vi "Range test.vi"() -> ()   [LabVIEW 2019]
uses:
  <userlib>/Agilent34410A/Agilent34410A DMM_Func.ctl
panel:
  out "Function Range Out":u16(ring) items=["100 mV", "1 V", "10 V", "100 V", "1000 V", "Min", "Max", "Def"]
  in  "error in (no error)":errorcluster
  out "Range Value":dbl
  out "Autorange":bool
  out "ChaineRep":string caption="Chaîne de réponse"
  in  "Set":bool
  out "ChaineCom":string caption="Chaîne de commande"
  in  "Function Range":u16(ring) items=["100 Ohms", "1 kOhms", "10 kOhms", "100 kOhms", "1 MOhms", "10 MOhms", "100 MOhms", "1 GOhms", "Min", "Max", "Def"]
  in  "DMM Function":T1
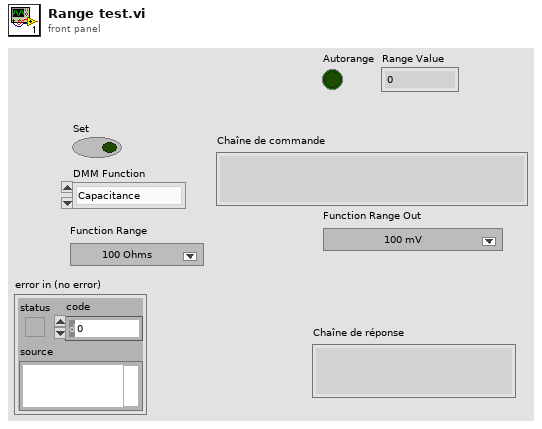
[diagram p1: front panel]
types:
  T1 = typedef "Agilent34410A DMM_Func.ctl" = enum16{"Capacitance", "Continuity", "Current AC", "Current", "Diode", "Frequency", "4W Resistance", "Period", "Resistance", "Temperature", "Voltage AC", "Voltage"}
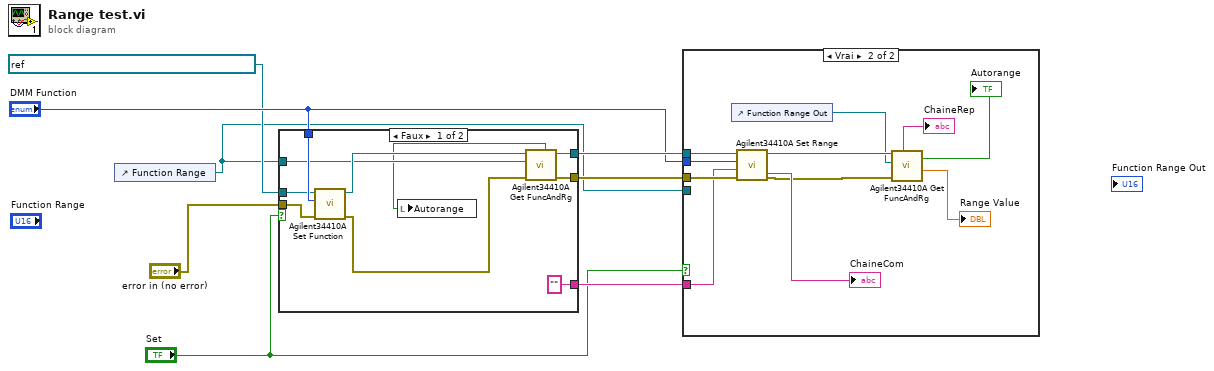
[diagram p0: block diagram]
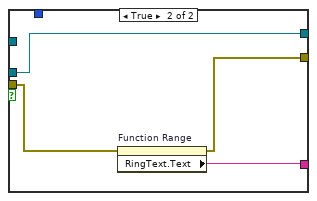
[diagram p2: hidden frame]
diagram:
  n1 = control-ref of="Function Range"() -> (w1:refnum<vi>)
  n2 = case shown="Faux" "Set" {
    tunnel: [w18 w19] -> w8
    tunnel: [w17 w22] -> w7
    tunnel: ["" ("RingText.Text") w21] -> w6
    tunnel: "DMM Function" -> [w16 _]
    tunnel: refnum<visa-resource-name> "USB0::0x0957::0x0607::MY47021456::INSTR" ("VISA Rsrc") -> [w15 w22]
    tunnel: "error in (no error)" -> [w13 w20]
    tunnel: w1 -> [w12 _]
    frame False {
      n3 = call <userlib>:"Agilent34410A Set Function.vi"("error in (no error)"=w13, "DMM Function"=w16, "VISA Rsrc"=w15) -> ("error out"=w11:errorcluster, "VISA Rsrc Out"=w14:refnum<visa-resource-name>)  [unwired: 6 in, 1 out]
      n4 = call <userlib>:"Agilent34410A Get FuncAndRg.vi"("error in (no error)"=w11, "Refnum Cmde"=w12, "VISA Rsrc"=w14) -> ("error out"=w18:errorcluster, "VISA Rsrc Out"=w17:refnum<visa-resource-name>, "Autorange"=w9:bool)  [unwired: 1 in, 5 out]
      n5 = local write "Autorange"(w9) -> ()
    }
    frame True {
      n6 = property on="Function Range" class="MDér (strict)"(error in=w20) -> (error out=w19:errorcluster, "RingText.Text"=w21:string)  [unwired: 1 in, 1 out]
    }
  }
  n7 = case shown="Vrai" "Set" {
    tunnel: w8 -> [_ w33]
    tunnel: w7 -> [_ w32]
    tunnel: "DMM Function" -> [_ w30]
    tunnel: w6 -> [_ w29]
    tunnel: w1 -> [_ _]
    frame False {
    }
    frame True {
      n8 = control-ref of="Function Range Out"() -> (w23:refnum<vi>)
      n9 = call <userlib>:"Agilent34410A Set Range.vi"("error in (no error)"=w33, "Range String"=w29, "DMM Function"=w30, "VISA Rsrc"=w32) -> ("error out"=w28:errorcluster, "VISA Rsrc Out"=w27:refnum<visa-resource-name>, "ChaineCom"=→"ChaineCom":string)  [unwired: 5 in]
      n10 = call <userlib>:"Agilent34410A Get FuncAndRg.vi"("error in (no error)"=w28, "Refnum Cmde"=w23, "VISA Rsrc"=w27) -> ("Range Value"=→"Range Value":dbl, "Autorange"=→"Autorange":bool, "ChaineRep"=→"ChaineRep":string)  [unwired: 1 in, 5 out]
    }
  }
